vi "EncodeMaskedBytes.vi"(8 "error in (no error)":errorcluster, 11 "Raw Data":u8[](array[numeric])) -> (0 "error out":errorcluster, 3 "Masked Data":u8[](array[numeric]))   [LabVIEW 2021, in "WebSockets.lvlib" / "WebSocket.lvclass"]
doc: "Unmasks incoming data. Data sent to the client does not need to be masked.\nWebSockets 2.0.1.40\nSam Sharp - MediaMongrels Ltd\nCopyright (c) 2019, MediaMongrels Ltd"
uses:
  WebSocket.lvclass
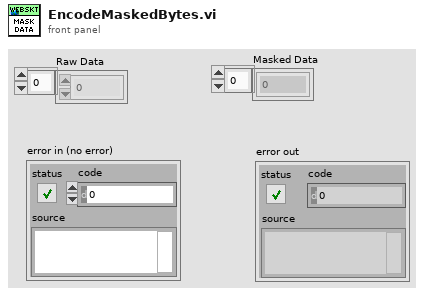
[diagram p1: front panel]
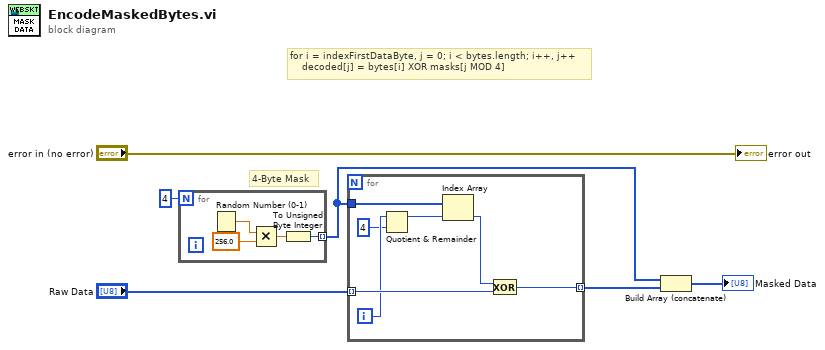
[diagram p0: block diagram]
diagram:
  # "4-Byte Mask"
  # "for i = indexFirstDataByte, j = 0; i < bytes.length; i++, j++\n    decoded[j] = bytes[i] XOR masks[j MOD 4]"
  n1 = for {
    N: 4 -> [_]
    tunnel: [w7] -> w2 mode=indexing
    n2 = Random Number (0-1)() -> (number: 0 to 1=w10:dbl)
    n3 = Multiply(x=w10, y=256.0) -> (x*y=w8:dbl)
    n4 = To Unsigned Byte Integer(number=w8) -> (unsigned 8bit integer=w7:u8)
  }
  n5 = for {
    tunnel: "Raw Data" -> [w17] mode=indexing
    tunnel: w2 -> [w13]
    tunnel: [w11] -> w1 mode=indexing
    i -> [w16]
    n6 = Quotient & Remainder(x=w16, y=4) -> (x-y*floor(x/y)=w14:i32)  [unwired: 1 out]
    n7 = Index Array(array=w13, index=w14) -> (element=w12:u8)
    n8 = Exclusive Or(1:w17, 2:w12) -> (0:w11:u8)
  }
  n9 = Build Array (concatenate)(w2, w1) -> (→"Masked Data":u8[])
  "error out" <- "error in (no error)"
